vi "rad_Refresh Target Information.vi"(5 "Password":string, 7 "Reduce Discovery Timeout":bool=TRUE, 8 "error in (no error)":errorcluster, 10 "User Added Targets Only":bool, 11 "User Added Targets":string[](array[string])) -> (0 "error out":errorcluster, 3 "Targets Information":T1[](array[typedef]) {"Primary NIC"."IP Address Request Mode" items=["Static"=1, "DHCP/Link-Local"=2, "Link-Local Only"=4, "DHCP Only"=8]})   [LabVIEW 2020]
uses:
  TypeDefs/rad_Target Information.ctl
  TypeDefs/rad_Target Network Settings.ctl
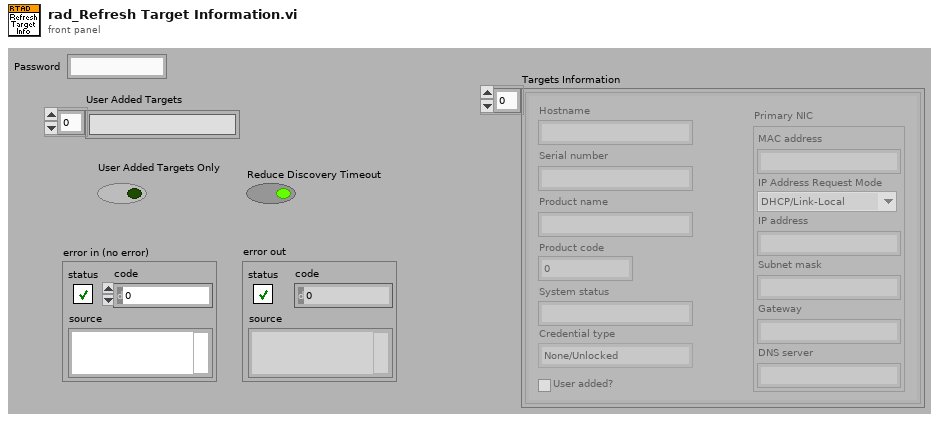
[diagram p1: front panel]
types:
  T1 = typedef "rad_Target Information.ctl" = cluster{"Hostname":string, "Serial number":string, "Product name":string, "Product code":i32, "System status":string, "Credential type":enum16{"None/Unlocked", "FTP Password", "NIAuth Credentials"}, "User added?":bool, "Primary NIC":T2}
  T2 = typedef "rad_Target Network Settings.ctl" = cluster{"MAC address":string, "IP Address Request Mode":i32, "IP address":string, "Subnet mask":string, "Gateway":string, "DNS server":string}
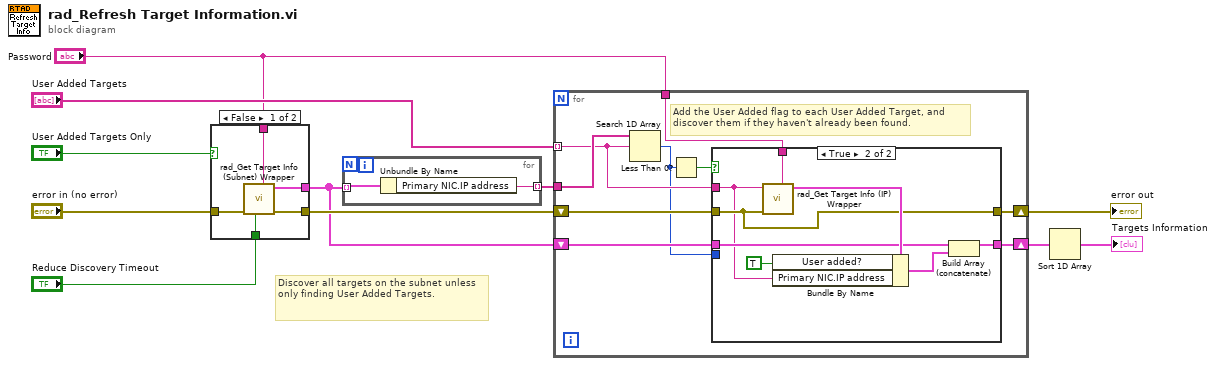
[diagram p0: block diagram]
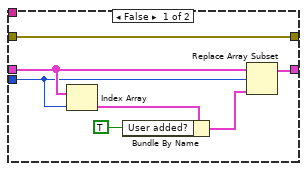
[diagram p2: hidden frame]
diagram:
  # "Discover all targets on the subnet unless only finding User Added Targets."
  n1 = case shown="False" "User Added Targets Only" {
    tunnel: "error in (no error)" -> [w16 w17]
    tunnel: [w15 _] -> w6
    tunnel: [w14 w17] -> w9
    tunnel: "Reduce Discovery Timeout" -> [w13 _]
    tunnel: "Password" -> [w12 _]
    frame False {
      n2 = call "rad_Get Target Info (Subnet) Wrapper.vi"("Password"=w12, "reduce discovery timeout (T)"=w13, "error in (no error)"=w16) -> ("error out"=w14:errorcluster, "target information"=w15:T1[])  [unwired: 7 in]
    }
    frame True {
    }
  }
  n3 = for {
    tunnel: w6 -> [w19] mode=indexing
    tunnel: [w18] -> w7 mode=indexing
    n4 = Unbundle By Name(w19) -> ("Primary NIC.IP address"=w18:string)
  }
  n5 = for {
    tunnel: "User Added Targets" -> [w25] mode=indexing
    tunnel: w7 -> [w27]
    shift-right: [w22] -> w5
    shift-left: w6 -> [w24]
    shift-right: [w21] -> w4
    shift-left: w9 -> [w28]
    tunnel: "Password" -> [w20]
    # "Add the User Added flag to each User Added Target, and discover them if they haven't already been found."
    n6 = Search 1D Array(1D array=w27, element=w25) -> (index of element=w23:i32)  [unwired: 1 in]
    n7 = Less Than 0?(x=w23) -> (x < 0?=w26:bool)
    n8 = case shown="True" w26 {
      tunnel: w28 -> [w35 w38]
      tunnel: w25 -> [_ w37]
      tunnel: [w35 w38] -> w21
      tunnel: w24 -> [w32 w40]
      tunnel: w23 -> [w29 _]
      tunnel: [w31 w39] -> w22
      tunnel: w20 -> [_ w36]
      frame False {
        n9 = Index Array(array=w32, index=w29) -> (element=w34:T1)
        n10 = Bundle By Name(cluster=w34, "User added?"=TRUE ("User Added?")) -> (w30:T1)
        n11 = Replace Array Subset(array=w32, new element=w30, index=w29) -> (w31:T1[])
      }
      frame True {
        n12 = call "rad_Get Target Info (IP) Wrapper.vi"("Password"=w36, "error in (no error)"=w38, "target address"=w37) -> ("Target settings"=w43:T1)  [unwired: 7 in, 1 out]
        n13 = Bundle By Name(cluster=w43, "User added?"=TRUE ("User Added?"), "Primary NIC.IP address"=w37) -> (w41:T1)
        n14 = Build Array (concatenate)(w40, w41) -> (w39:T1[])
      }
    }
  }
  "error out" <- w4
  n15 = Sort 1D Array(array=w5) -> (sorted array=→"Targets Information":T1[])
